vi "SaveSXM (SubVI).vi"(0 "Application ref in":refnum<vi>, 1 "seconds since 1Jan1904":timestamp, 2 "DataIn":dbl[][][](array[numeric]), 3 "error in (no error)":errorcluster, 4 "Channels indexes (0-23)":i32[](array[numeric]), 5 "selected path":path) -> (7 "Application ref out":refnum<vi>, 10 "error out":errorcluster)   [LabVIEW 2014]
uses:
  <userlib>/Nanonis Prog Interface V5/Nanonis Prog Interface.lvlib
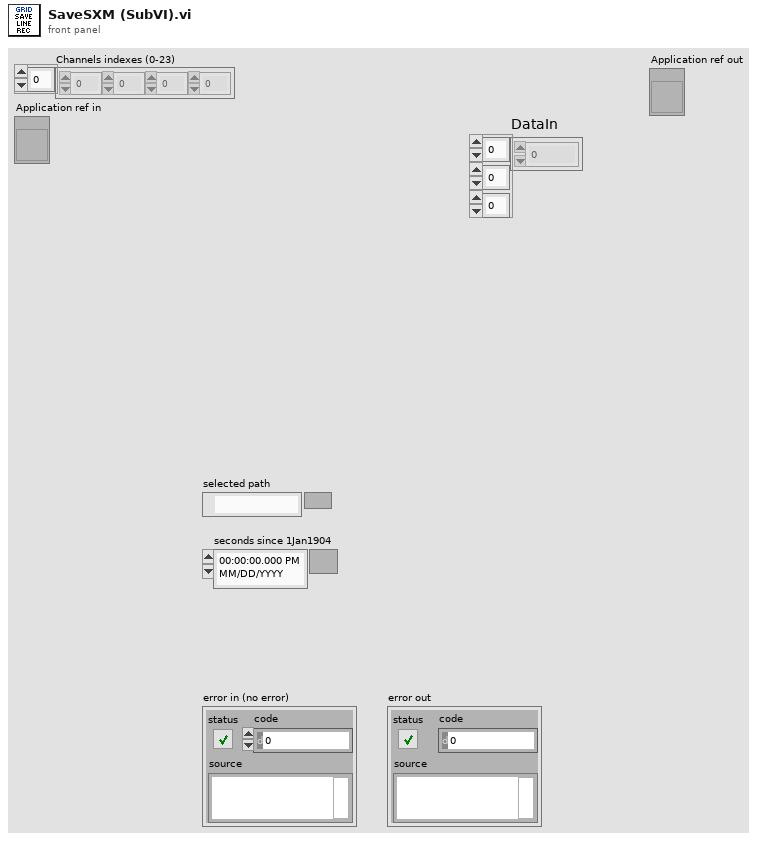
[diagram p1: front panel]
types:
  T1 = cluster{"center X":sgl, "center Y":sgl, "angle":sgl, "width":sgl, "height":sgl, "# pixels":i32, "# lines":i32}
  T2 = cluster{"Name":string, "Calibration":sgl, "Offset":sgl, "Channel index":i32}[]
  T3 = cluster{"up/down":bool, "time/line":sgl, "start time":timestamp, "end time":timestamp}
  T4 = cluster{"Name":string, "Calibration":sgl, "Offset":sgl, "Channel index":i32}
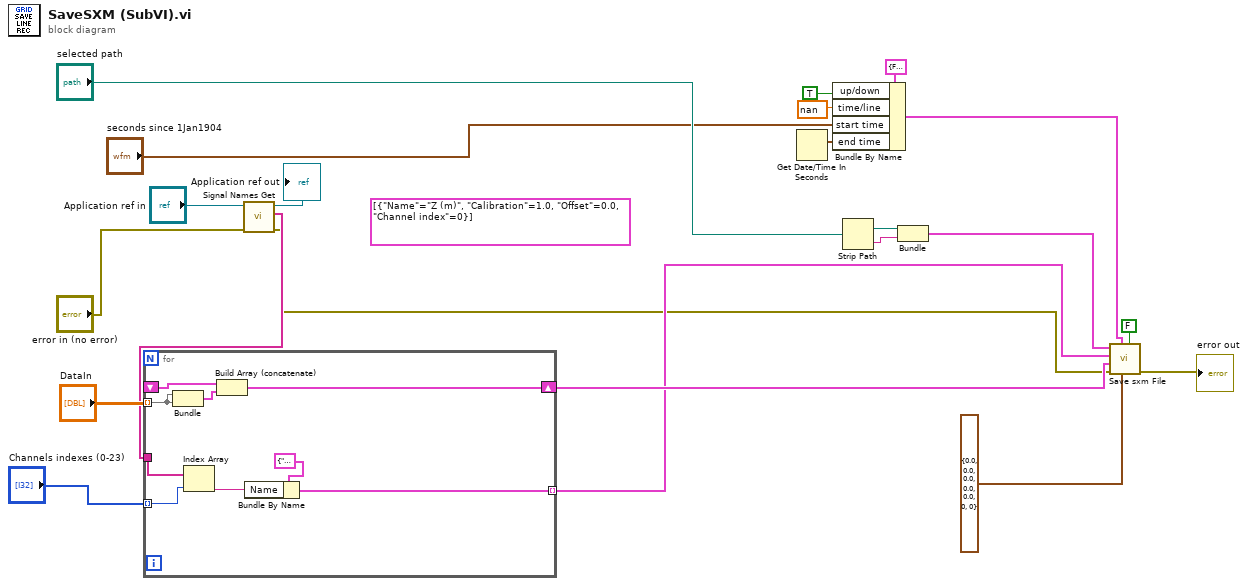
[diagram p0: block diagram]
diagram:
  (unwired) T2 [{"Name"="Z (m)", "Calibration"=1.0, "Offset"=0.0, "Channel index"=0}] ("Channels config")
  n1 = call <userlib>:"Signal Names Get.vi"("error in (no error)"="error in (no error)", "Application ref in"="Application ref in") -> ("error out"=w3:errorcluster, "Signals Names"=w7:string[], "Application ref out"=→"Application ref out":refnum<vi>)  [unwired: 5 in]
  n2 = for {
    tunnel: "DataIn" -> [w31] mode=indexing
    shift-right: [w29] -> w8
    shift-left: _ -> [w28]
    tunnel: w7 -> [w27]
    tunnel: [w25] -> w6 mode=indexing
    tunnel: "Channels indexes (0-23)" -> [w23] mode=indexing
    n3 = Bundle("DataIn"=w31, "DataIn"=w31) -> (w30:cluster{"DataIn":dbl[][], "DataIn":dbl[][]})  [unwired: 1 in]
    n4 = Index Array(array=w27, index=w23) -> (element=w24:string)
    n5 = Build Array (concatenate)(w28, w30) -> (w29:cluster{"DataIn":dbl[][], "DataIn":dbl[][]}[])
    n6 = Bundle By Name(cluster=T4 {"Name"="Z (m)", "Calibration"=1.0, "Offset"=0.0, "Channel index"=0} ("channel config"), "Name"=w24) -> (w25:T4)
  }
  n7 = Get Date/Time In Seconds() -> (seconds since 1Jan1904=w16:timestamp)
  n8 = Bundle By Name(cluster=T3 {"up/down"=FALSE, "time/line"=0.0, "start time"=timestamp(0 s since 1904-01-01), "end time"=timestamp(0 s since 1904-01-01)} ("Scan param"), "up/down"=TRUE, "time/line"=sgl nan ("input 7"), "start time"="seconds since 1Jan1904", "end time"=w16) -> (w15:T3)
  n9 = Strip Path(path="selected path") -> (stripped path=w18:path, name=w19:string)
  n10 = Bundle("stripped path"=w18, "name"=w19) -> (w20:cluster{"stripped path":path, "name":string})  [unwired: 1 in]
  n11 = call <userlib>:"Save sxm File.vi"("Auto file naming? (T)"=FALSE, "Scanfield"=T1 {"center X"=0.0, "center Y"=0.0, "angle"=0.0, "width"=0.0, "height"=0.0, "# pixels"=0, "# lines"=0}, "Scan param"=w15, "error in (no error)"=w3, "Channels data"=w8, "Channels config"=w6, "Filename control"=w20) -> ("error out"=→"error out":errorcluster)  [unwired: 2 in, 2 out]
